vi "Read Measurement (List Sweep).vi"(0 "VISA resource name":refnum<visa-resource-name>, 5 "Timeout (10000 ms)":i32=10000 format="%.0g", 11 "error in (no error)":errorcluster) -> (4 "VISA resource name out":refnum<visa-resource-name>, 6 "Measurement Data":dbl[](array[numeric]), 15 "error out":errorcluster)   [LabVIEW 2014, in "Agilent MXA Series.lvlib"]
doc: "Reads the measurement result from the spectrum analyzer(List Sweep) ."
uses:
  Agilent MXA Series.lvlib
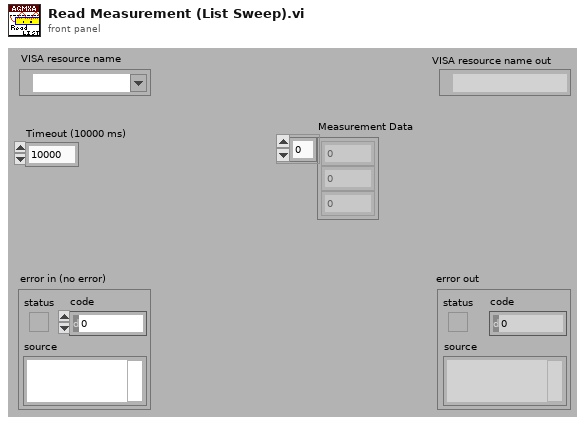
[diagram p1: front panel]
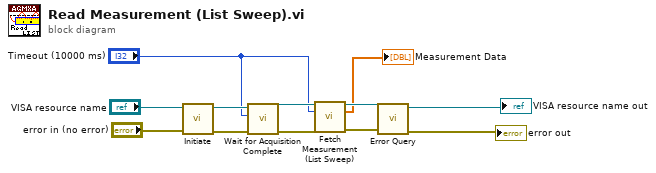
[diagram p0: block diagram]
diagram:
  n1 = call "Initiate.vi"("error in (no error)"="error in (no error)", "VISA resource name"="VISA resource name") -> ("error out"=w9:errorcluster, "VISA resource name out"=w10:refnum<visa-resource-name>)  [unwired: 8 in]
  n2 = call "Wait for Acquisition Complete.vi"("error in (no error)"=w9, "Maximum Time (10000)"="Timeout (10000 ms)", "VISA resource name"=w10) -> ("error out"=w7:errorcluster, "VISA resource name out"=w8:refnum<visa-resource-name>)  [unwired: 7 in]
  n3 = call "Fetch Measurement (List Sweep).vi"("VISA resource name"=w8, "Timeout (10000 ms)"="Timeout (10000 ms)", "error in (no error)"=w7) -> ("VISA resource name out"=w6:refnum<visa-resource-name>, "Measurement Data"=→"Measurement Data":dbl[], "error out"=w5:errorcluster)  [unwired: 10 in]
  n4 = call "Error Query.vi"("error in (no error)"=w5, "VISA resource name"=w6) -> ("error out"=→"error out":errorcluster, "VISA resource name out"=→"VISA resource name out":refnum<visa-resource-name>)  [unwired: 6 in, 2 out]
